vi "ex_CreateSignalChunkStringSub.vi"(5 "data":string[](array[string]), 6 "Signals":waveform(dbl)[](array[waveform]), 7 "format":string[](array[string])) -> (0 "Array":string[][](array[string]))   [LabVIEW 2020]
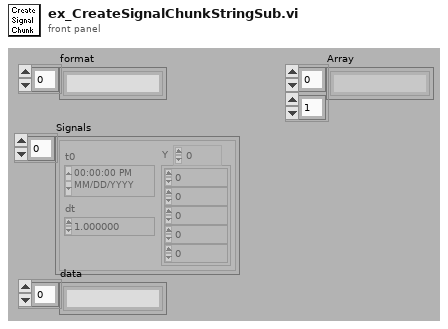
[diagram p1: front panel]
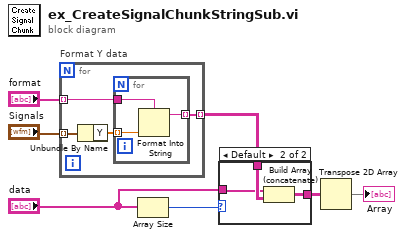
[diagram p0: block diagram]
diagram:
  n1 = for "Format Y data" {
    tunnel: "Signals" -> [w10] mode=indexing
    tunnel: [w9] -> w6 mode=indexing
    tunnel: "format" -> [w8] mode=indexing
    n2 = Unbundle By Name(w10) -> ("Y"=w11:dbl[])
    n3 = for {
      tunnel: [w12] -> w9 mode=indexing
      tunnel: w11 -> [w14] mode=indexing
      tunnel: w8 -> [w13]
      n4 = Format Into String(format string=w13, w14) -> (resulting string=w12:string)  [unwired: 2 in, 1 out]
    }
  }
  n5 = Array Size(array="data") -> (size(s)=w4:i32)
  n6 = case shown="Default" w4 {
    tunnel: [w15 w18] -> w2
    tunnel: w6 -> [w15 w17]
    tunnel: "data" -> [_ w16]
    frame 0 {
    }
    frame Default {
      n7 = Build Array (concatenate)(w16, w17) -> (w18:string[][])
    }
  }
  n8 = Transpose 2D Array(2D array=w2) -> (transposed array=→"Array":string[][])
